vi "LuaVIEW Loaded Function Infos_srv.vi"(7 "certificate":string) -> (8 "function infos":T1[](array[typedef]), 15 "error out":errorcluster)   [LabVIEW 2012]
doc: "Collects a list of info clusters of the LuaVIEW function VIs that are loaded on the server. Usually, loaded function VIs will have been registered as public functions. The docstrings and synopses are excluded from the collected info clusters."
uses:
  typedefs/clusters/LuaVIEW Function Info.ctl
  clientsrv/typedefs/t_ClientSrv Access Levels.ctl
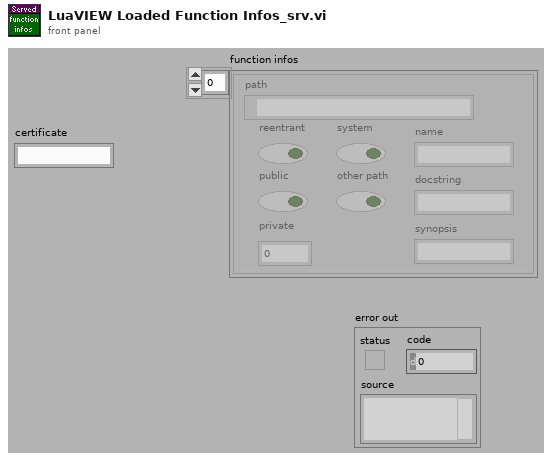
[diagram p1: front panel]
types:
  T1 = typedef "LuaVIEW Function Info.ctl" = cluster{"path":path, "reentrant":bool, "public":bool, "private":i32, "system":bool, "other path":bool, "name":string, "docstring":string, "synopsis":string}
  T2 = typedef "t_ClientSrv Access Levels.ctl" = enum16{"observer", "operator", "local"}
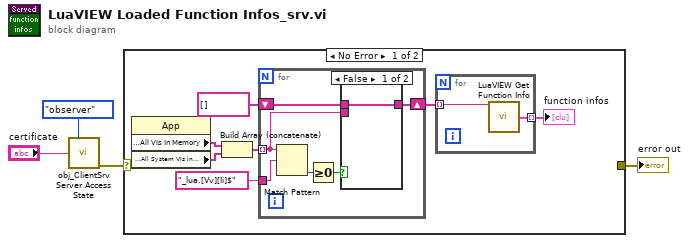
[diagram p0: block diagram]
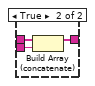
[diagram p2: hidden frame]
diagram:
  n1 = call "obj_ClientSrv Server Access State.vi"("access level"=t_ClientSrv_Access_Levels."observer", "certificate in"="certificate") -> ("error out"=w2:errorcluster)  [unwired: 11 in, 2 out]
  n2 = case shown="No Error" w2 {
    selector: w2 -> [_ w24]
    tunnel: [_ w24] -> w1
    frame No Error {
      n3 = property class="App"() -> ("Application:All VIs In Memory"=w6:string[], "Application:All System VIs in Memory"=w5:string[])  [unwired: 2 in, 2 out]
      n4 = Build Array (concatenate)(w6, w5) -> (w7:string[])
      n5 = for {
        tunnel: w7 -> [w15] mode=indexing
        tunnel: "_lua.[Vv][Ii]$" -> [w19]
        shift-right: [w14] -> w9
        shift-left: string[] [] -> [w16]
        n6 = Match Pattern(string=w15, regular expression=w19) -> (offset past match=w18:i32)  [unwired: 1 in, 3 out]
        n7 = Greater Or Equal To 0?(x=w18) -> (x >= 0?=w17:bool)
        n8 = case shown="False" w17 {
          tunnel: w16 -> [w20 w23]
          tunnel: w15 -> [_ w22]
          tunnel: [w20 w21] -> w14
          frame False {
          }
          frame True {
            n9 = Build Array (concatenate)(w23, w22) -> (w21:string[])
          }
        }
      }
      n10 = for {
        tunnel: w9 -> [w12] mode=indexing
        tunnel: [w13] -> w8 mode=indexing
        n11 = call "LuaVIEW Get Function Info.vi"("function VI name (use path)"=w12) -> ("function info"=w13:T1)  [unwired: 13 in, 1 out]
      }
      "function infos" <- w8
    }
    frame Error {
    }
  }
  "error out" <- w1
